vi "IEEE754_schreiben.vi"(11 "Wert":sgl) -> (0 "lo":u16, 3 "hi":u16)   [LabVIEW 2020, in "ABB-EL3000.lvlib" / "Allgemeine VI.lvlib"]
uses:
  Allgemeine VI.lvlib
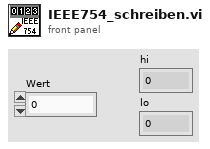
[diagram p1: front panel]
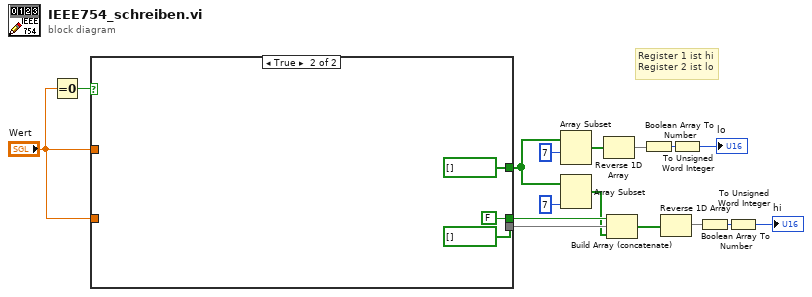
[diagram p0: block diagram]
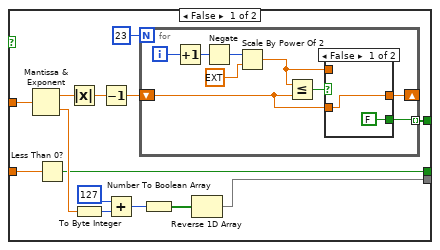
[diagram p2: hidden frame]
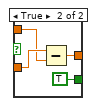
[diagram p3: hidden frame]
diagram:
  # "Register 1 ist hi\nRegister 2 ist lo"
  n1 = Equal To 0?(x="Wert") -> (x = 0?=w1:bool)
  n2 = case shown="True" w1 {
    tunnel: [w25 FALSE] -> w16
    tunnel: [w24 bool[] []] -> w15
    tunnel: [w19 bool[] []] -> w14
    tunnel: "Wert" -> [w18 _]
    tunnel: "Wert" -> [w17 _]
    frame False {
      n3 = Mantissa & Exponent(0:w17) -> (1:w22:sgl, 2:w30:sgl)
      n4 = Less Than 0?(x=w18) -> (x < 0?=w25:bool)
      n5 = Absolute Value(x=w22) -> (abs(x)=w21:sgl)
      n6 = To Byte Integer(number=w30) -> (8bit integer=w29:i8)
      n7 = Decrement(x=w21) -> (x-1=w20:sgl)
      n8 = Add(x=i8 127, y=w29) -> (x+y=w27:i8)
      n9 = for {
        N: 23 -> [_]
        shift-right: [w32] -> _
        shift-left: w20 -> [w33]
        tunnel: [w31] -> w19 mode=indexing
        i -> [w39]
        n10 = Increment(x=w39) -> (x+1=w38:i32)
        n11 = Negate(x=w38) -> (-x=w37:i32)
        n12 = Scale By Power Of 2(n=w37, x=ext 1.0) -> (x*2^n=w34:ext)
        n13 = Less Or Equal?(x=w34, y=w33) -> (x <= y?=w35:bool)
        n14 = case shown="False" w35 {
          tunnel: w34 -> [_ w44]
          tunnel: w33 -> [w41 w45]
          tunnel: [w41 w43] -> w32
          tunnel: [FALSE TRUE] -> w31
          frame False {
          }
          frame True {
            n15 = Subtract(x=w45, y=w44) -> (x-y=w43:ext)
          }
        }
      }
      n16 = Number To Boolean Array(number=w27) -> (Boolean array=w26:bool[])
      n17 = Reverse 1D Array(array=w26) -> (reversed array=w24:bool[])
    }
    frame True {
    }
  }
  n18 = Array Subset(array=w14, index=7 ("Index")) -> (w12:bool[])  [unwired: 1 in]
  n19 = Array Subset(array=w14, length=7 ("Länge")) -> (w8:bool[])  [unwired: 1 in]
  n20 = Reverse 1D Array(array=w12) -> (reversed array=w11:bool[])
  n21 = Build Array (concatenate)(w16, w15, w8) -> (w7:bool[])
  n22 = Boolean Array To Number(Boolean array=w11) -> (number=w10:u32)
  n23 = Reverse 1D Array(array=w7) -> (reversed array=w5:bool[])
  n24 = To Unsigned Word Integer(number=w10) -> (unsigned 16bit integer=→"lo":u16)
  n25 = Boolean Array To Number(Boolean array=w5) -> (number=w6:u32)
  n26 = To Unsigned Word Integer(number=w6) -> (unsigned 16bit integer=→"hi":u16)
